vi "Tx.vi"(8 "error in (no error)":errorcluster, 10 "Command Parameters":T1, 11 "Dispatcher in":refnum<class "Dispatcher Thread.lvclass">) -> (0 "error out":errorcluster, 3 "Dispatcher out":refnum<class "Dispatcher Thread.lvclass">)   [LabVIEW 2020, in "DSF Core.lvlib" / "Dispatcher Thread.lvclass"]
uses:
  Dispatcher Thread.lvclass
  Interface/Plugin/Command.ctl
  Interface/Plugin/Plugin Interface.lvclass
  Interface/Dispatcher/Rx Parameters.ctl
  Interface/Dispatcher/Dispatcher Interface.lvclass
  Interface/Dispatcher/Parameters.ctl
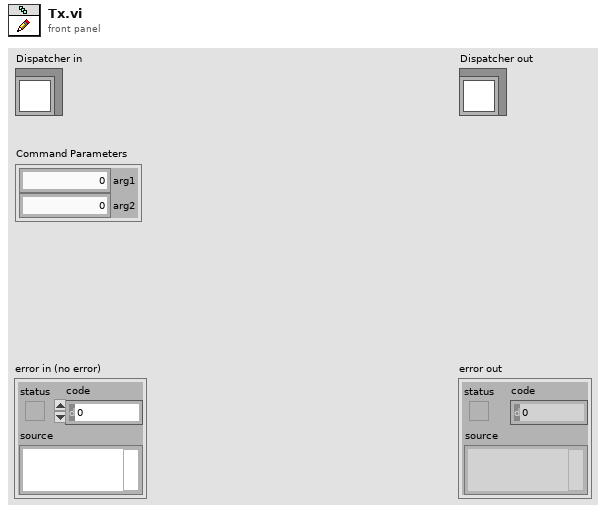
[diagram p1: front panel]
types:
  T1 = typedef "DSF Core.lvlib/Dispatcher Interface.lvclass/Parameters.ctl" = cluster{"arg1":u64, "arg2":u64}
  T2 = typedef "DSF Core.lvlib/Plugin Interface.lvclass/Command.ctl" = enum8{"Idle", "Start", "Set Inline Buffer", "Rx", "Tx", "Shutdown", "Error"}
  T3 = typedef "DSF Core.lvlib/Dispatcher Interface.lvclass/Rx Parameters.ctl" = cluster{"Plugin ID":u8, "Transfer Group ID":u8, "unused long":u16, "Late Count":i32, "Iteration":u64}
  T4 = typedef "DSF Core.lvlib/Dispatcher Thread.lvclass/Plugin Settings.ctl" = cluster{"Transfer Group threads":i32[], "Plugin Thread Interfaces":refnum<class "Plugin Interface.lvclass">[]}
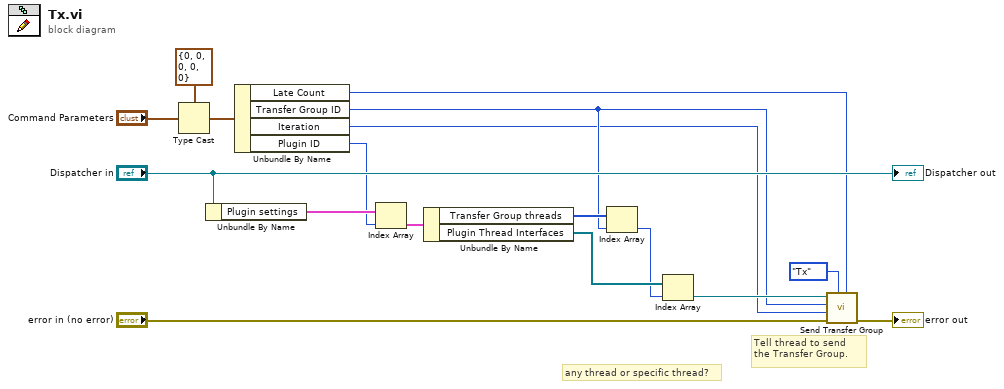
[diagram p0: block diagram]
diagram:
  # "any thread or specific thread?"
  # "Tell thread to send the Transfer Group."
  n1 = Type Cast(type=T3 {"Plugin ID"=0, "Transfer Group ID"=0, "unused long"=0, "Late Count"=0, "Iteration"=0}, x="Command Parameters") -> (*(type *) &x=w15:T3)
  n2 = Unbundle By Name("Dispatcher in") -> ("Plugin settings"=w14:T4[])
  n3 = Unbundle By Name(w15) -> ("Late Count"=w3:i32, "Transfer Group ID"=w5:u8, "Iteration"=w4:u64, "Plugin ID"=w12:u8)
  n4 = Index Array(array=w14, index=w12) -> (element=w9:T4)
  n5 = Unbundle By Name(w9) -> ("Transfer Group threads"=w8:i32[], "Plugin Thread Interfaces"=w2:refnum<class "Plugin Interface.lvclass">[])
  n6 = Index Array(array=w8, index=w5) -> (element=w1:i32)
  n7 = Index Array(array=w2, index=w1) -> (element=w7:refnum<class "Plugin Interface.lvclass">)
  n8 = call "Send Transfer Group.vi"("Late Count"=w3, "Command"=Command."Tx", "error in (no error)"="error in (no error)", "Transfer Group iteration"=w4, "Transfer Group ID"=w5, "Plugin Interface in"=w7) -> ("error out"=→"error out":errorcluster)  [unwired: 4 in, 1 out]
  "Dispatcher out" <- "Dispatcher in"
